vi "Parse Frame string.vi"(3 "frame string":string) -> (0 "Parse OK":bool, 1 "output cluster":T1 {"Data" format="%.0x"; "ID" format="%.0x"})   [LabVIEW 2021, in "uCanDriver.lvlib" / "uCAN.lvclass"]
uses:
  uCAN.lvclass
  typedefs/frame.ctl
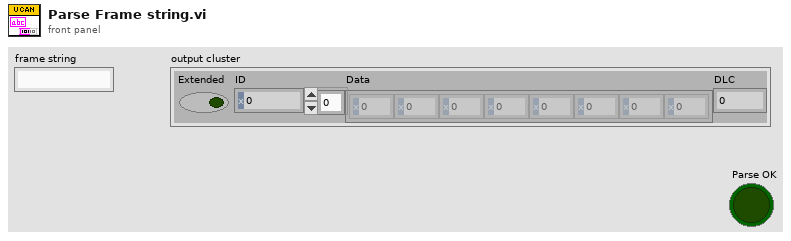
[diagram p1: front panel]
types:
  T1 = typedef "uCanDriver.lvlib/uCAN.lvclass/frame.ctl" = cluster{"Extended":bool, "ID":u32, "Data":u8[], "DLC":u8}
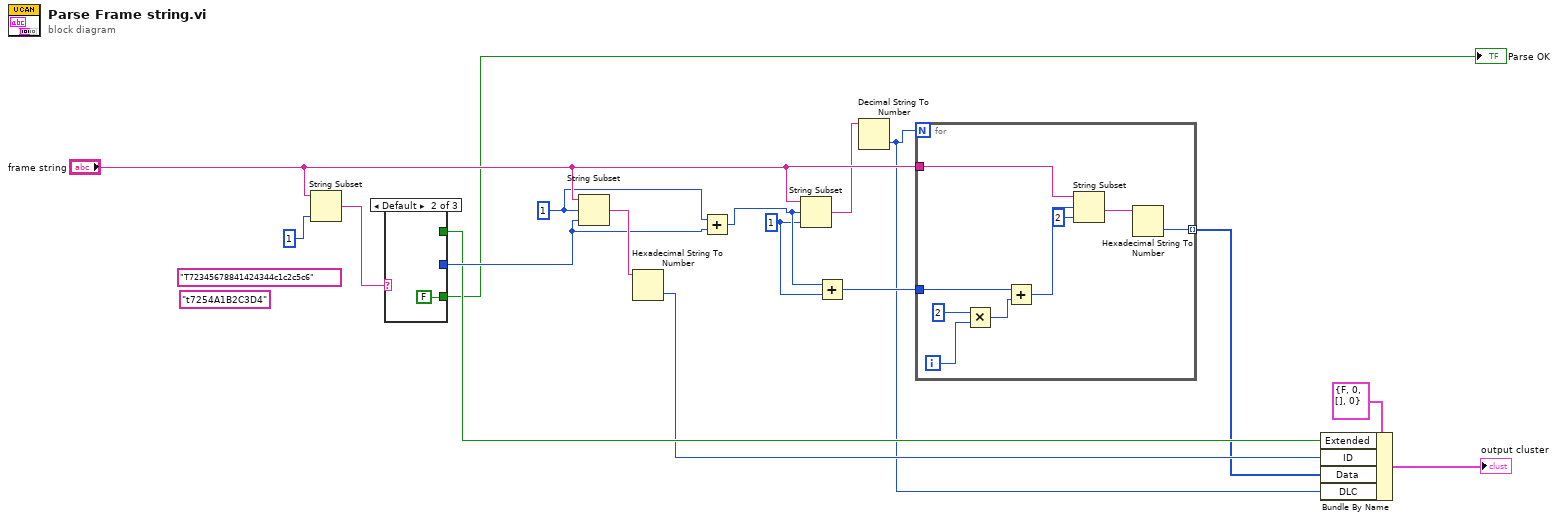
[diagram p0: block diagram]
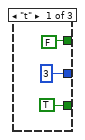
[diagram p2: hidden frame]
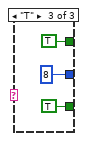
[diagram p3: hidden frame]
diagram:
  (unwired) "T72345678841424344c1c2c5c6"
  w8 = 1 ("length (rest)")
  w12 = 1 ("offset (0)")
  (unwired) "t7254A1B2C3D4"
  n1 = String Subset(string="frame string", length (rest)=1 ("length (rest)")) -> (substring=w14:string)  [unwired: 1 in]
  n2 = case shown="Default" w14 {
    tunnel: [3 ("offset (0)") _ 8 ("offset (0)")] -> w11
    tunnel: [FALSE _ TRUE] -> w5
    tunnel: [TRUE FALSE TRUE] -> w1
    frame "t" {
    }
    frame Default {
    }
    frame "T" {
    }
  }
  "Parse OK" <- w1
  n3 = String Subset(string="frame string", offset (0)=w12, length (rest)=w11) -> (substring=w13:string)
  n4 = Hexadecimal String To Number(string=w13) -> (number=w4:u32)  [unwired: 2 in, 1 out]
  n5 = Add(x=w12, y=w11) -> (x+y=w9:i32)
  n6 = String Subset(string="frame string", offset (0)=w9, length (rest)=w8) -> (substring=w10:string)
  n7 = Add(x=w9, y=w8) -> (x+y=w7:i32)
  n8 = Decimal String To Number(string=w10) -> (number=w2:i32)  [unwired: 2 in, 1 out]
  n9 = for {
    N: w2 -> [_]
    tunnel: w7 -> [w33]
    tunnel: "frame string" -> [w28]
    tunnel: [w26] -> w3 mode=indexing
    i -> [w31]
    n10 = Multiply(x=2, y=w31) -> (x*y=w32:i32)
    n11 = Add(x=w33, y=w32) -> (x+y=w29:i32)
    n12 = String Subset(string=w28, offset (0)=w29, length (rest)=2 ("length (rest)")) -> (substring=w27:string)
    n13 = Hexadecimal String To Number(string=w27) -> (number=w26:u32)  [unwired: 2 in, 1 out]
  }
  n14 = Bundle By Name(cluster=T1 {"Extended"=FALSE, "ID"=0, "Data"=[], "DLC"=0} ("Frame"), "Extended"=w5, "ID"=w4, "Data"=w3, "DLC"=w2) -> (→"output cluster":T1)
